vi "IT-M3400 Battery Charge&Discharge Test.vi"() -> ()   [LabVIEW 2020]
doc: "The example's main function is: set the charge or discharge mode of the relevant parameters, and run"
uses:
  IT-M3400.lvlib
panel:
  in  "Serial Configuration":T1={"Baud Rate"=9600, "Parity"=0, "Data Bits"=8, "Stop Bits"=10, "Flow Control"=0} {"Flow Control" items=["None", "XON/XOFF", "RTS/CTS", "XON/XOFF & RTS/CTS", "DTR/DSR", "XON/XOFF & DTR/DSR"]; "Stop Bits" items=["1.0"=10, "1.5"=15, "2.0"=20]; "Data Bits" items=["7"=7, "8"=8]; "Parity" items=["None", "Odd", "Even", "Mark", "Space"]; "Baud Rate" items=["300"=300, "600"=600, "1200"=1200, "2400"=2400, "4800"=4800, "9600"=9600, "19200"=19200]}
  out "error out":errorcluster
  out "VISA resource name out":refnum<visa-resource-name>
  in  "Battery File(1-10)":u8=1 min=1 max=10 step=1
  in  "Stop Time(s)":dbl
  in  "Stop Capacity(Ah)":dbl
  in  "Stop Current(A)":dbl
  in  "Stop Voltage(V)":dbl
  in  "Battery Mode":u8(ring) items=["Charge", "Discharge"]
  in  "Charge Current(A)":dbl
  in  "Charge Voltage(V)":dbl
  in  "Channel":i32(ring)=1 items=["Channel 1"=1, "Channel 2"=2, "Channel 3"=3, "Channel 4"=4, "Channel 5"=5, "Channel 6"=6, "Channel 7"=7, "Channel 8"=8, "Channel 8"=9, "Channel 10"=10, "Channel 11"=11, "Channel 12"=12, "Channel 13"=13, "Channel 14"=14, "Channel 15"=15, "Channel 16"=16]
  in  "error in (no error)":errorcluster caption="error in"
  in  "VISA resource name":refnum<visa-resource-name>
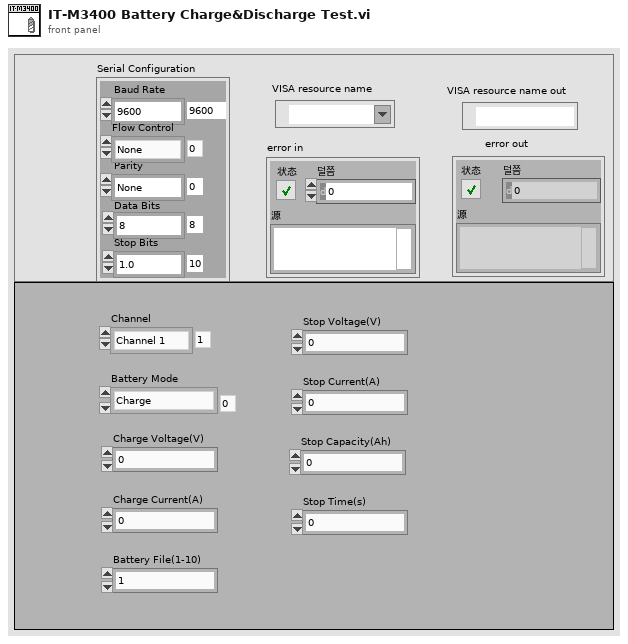
[diagram p1: front panel]
types:
  T1 = cluster{"Baud Rate":u32, "Parity":u16, "Data Bits":u16, "Stop Bits":u16, "Flow Control":u16}
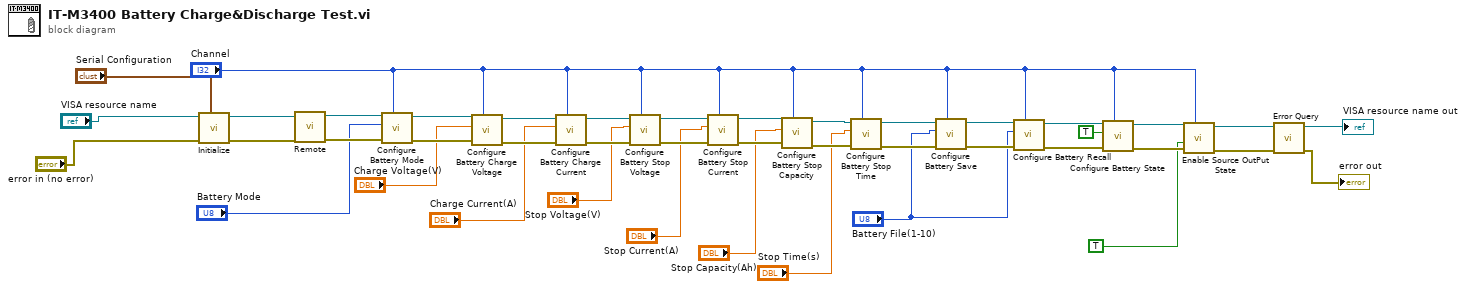
[diagram p0: block diagram]
diagram:
  n1 = call "Initialize.vi"("Serial Configuration"="Serial Configuration", "error in"="error in (no error)", "VISA resource name"="VISA resource name") -> ("error out"=w16:errorcluster, "VISA resource name out"=w17:refnum<visa-resource-name>)  [unwired: 7 in]
  n2 = call "Remote.vi"("error in"=w16, "VISA resource name"=w17) -> ("error out"=w41:errorcluster, "VISA resource name out"=w42:refnum<visa-resource-name>)  [unwired: 8 in]
  n3 = call "Configure Battery Mode.vi"("Channel"="Channel", "error in"=w41, "Battery Mode"="Battery Mode", "VISA resource name"=w42) -> ("error out"=w39:errorcluster, "VISA resource name out"=w40:refnum<visa-resource-name>)  [unwired: 6 in]
  n4 = call "Configure Battery Charge Voltage.vi"("Channel"="Channel", "error in"=w39, "Charge Voltage(V)"="Charge Voltage(V)", "VISA resource name"=w40) -> ("error out"=w37:errorcluster, "VISA resource name out"=w38:refnum<visa-resource-name>)  [unwired: 5 in]
  n5 = call "Configure Battery Charge Current.vi"("Channel"="Channel", "error in"=w37, "Charge Current(A)"="Charge Current(A)", "VISA resource name"=w38) -> ("error out"=w33:errorcluster, "VISA resource name out"=w34:refnum<visa-resource-name>)  [unwired: 6 in]
  n6 = call "Configure Battery Stop Voltage.vi"("Channel"="Channel", "error in"=w33, "Stop Voltage(V)"="Stop Voltage(V)", "VISA resource name"=w34) -> ("error out"=w31:errorcluster, "VISA resource name out"=w32:refnum<visa-resource-name>)  [unwired: 6 in]
  n7 = call "Configure Battery Stop Current.vi"("Channel"="Channel", "error in"=w31, "Stop Current(A)"="Stop Current(A)", "VISA resource name"=w32) -> ("error out"=w29:errorcluster, "VISA resource name out"=w30:refnum<visa-resource-name>)  [unwired: 6 in]
  n8 = call "Configure Battery Stop Capacity.vi"("Channel"="Channel", "error in"=w29, "Stop Capacity(Ah)"="Stop Capacity(Ah)", "VISA resource name"=w30) -> ("error out"=w27:errorcluster, "VISA resource name out"=w28:refnum<visa-resource-name>)  [unwired: 6 in]
  n9 = call "Configure Battery Stop Time.vi"("Channel"="Channel", "error in"=w27, "Stop Time(S)"="Stop Time(s)", "VISA resource name"=w28) -> ("error out"=w25:errorcluster, "VISA resource name out"=w26:refnum<visa-resource-name>)  [unwired: 6 in]
  n10 = call "Configure Battery Save.vi"("Channel"="Channel", "error in"=w25, "File"="Battery File(1-10)", "VISA resource name"=w26) -> ("error out"=w12:errorcluster, "VISA resource name out"=w13:refnum<visa-resource-name>)  [unwired: 6 in]
  n11 = call "Configure Battery Recall.vi"("Channel"="Channel", "error in"=w12, "File"="Battery File(1-10)", "VISA resource name"=w13) -> ("error out"=w10:errorcluster, "VISA resource name out"=w11:refnum<visa-resource-name>)  [unwired: 6 in]
  n12 = call "Configure Battery State.vi"("Channel"="Channel", "error in"=w10, "State"=TRUE, "VISA resource name"=w11) -> ("error out"=w7:errorcluster, "VISA resource name out"=w8:refnum<visa-resource-name>)  [unwired: 6 in]
  n13 = call "Enable Source OutPut State.vi"("Channel"="Channel", "error in"=w7, "State"=TRUE ("Enable Output|Intput"), "VISA resource name"=w8) -> ("error out"=w5:errorcluster, "VISA resource name out"=w6:refnum<visa-resource-name>)  [unwired: 6 in]
  n14 = call "Error Query.vi"("error in"=w5, "VISA resource name"=w6) -> ("error out"=→"error out":errorcluster, "VISA resource name out"=→"VISA resource name out":refnum<visa-resource-name>)  [unwired: 6 in, 2 out]
